vi "Save Tag Data to Database.vi"(7 "Database Connection":refnum<k7>, 8 "Error In":errorcluster) -> (0 "Error Out":errorcluster)   [LabVIEW 2019]
uses:
  SubVIs/WSData.vi
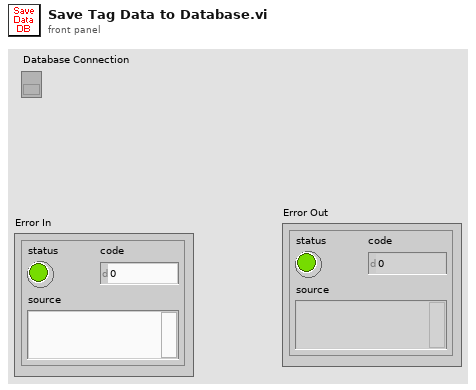
[diagram p1: front panel]
types:
  T1 = cluster{"TagId":string, "TagName":string, "TagType":string, "PhysicalChannel":tag, "Vmin":dbl, "Vmax":dbl, "Unit":string, "EUmin":dbl, "EUmax":dbl}[]
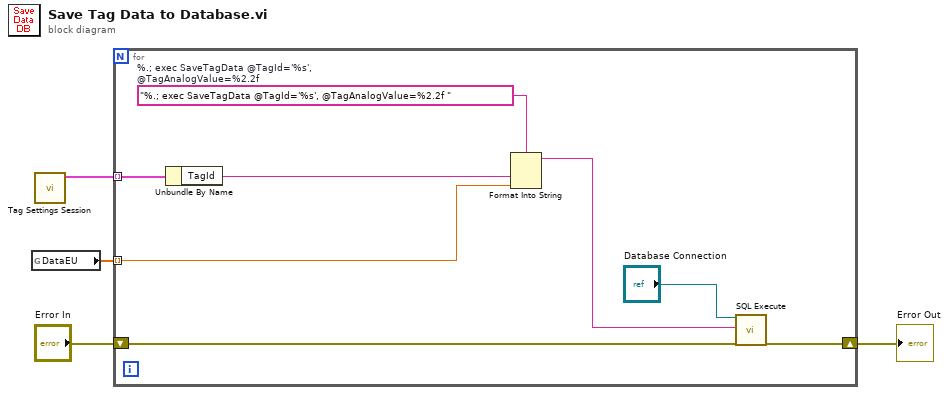
[diagram p0: block diagram]
diagram:
  n1 = global read "WSData.vi" "DataEU"() -> (w1:dbl[])
  n2 = call "Tag Settings Session.vi"() -> ("Tag Settings"=w2:T1)  [unwired: 10 in, 1 out]
  n3 = for {
    tunnel: w1 -> [w10] mode=indexing
    shift-right: [w11] -> w4
    shift-left: "Error In" -> [w12]
    tunnel: w2 -> [w6] mode=indexing
    w9 = "%.; exec SaveTagData @TagId='%s', @TagAnalogValue=%2.2f "  # %.; exec SaveTagData @TagId='%s', @TagAnalogValue=%2.2f
    n4 = Unbundle By Name(w6) -> ("TagId"=w5:string)
    n5 = Format Into String "Format Into String"(format string=w9, w5, w10) -> (resulting string=w8:string)  [unwired: 2 in, 1 out]
    n6 = call <vilib>:"SQL Execute.vi"("Connection In"="Database Connection", "SQL Query"=w8, "Error in (no error)"=w12) -> ("Error out"=w11:errorcluster)  [unwired: 15 in, 1 out]
  }
  "Error Out" <- w4
